vi "(Incomplete) Beta Function (obs).vi"(3 "a":dbl=nan format="%.2f", 4 "y":dbl format="%.2f", 5 "x":dbl format="%.2f") -> (2 "b(x, y, a)":dbl format="%.2f")   [LabVIEW 2020, in "NI_Gmath.lvlib"]
uses:
  NI_Gmath.lvlib
panel:
  # "This VI is obsolete !!!\nYou should replace this VI in your diagram with the \n(Incomplete) Beta Function VI.\n\nNOTE:   Please be aware that the new (Incomplete) Beta\n             Function VI is a polymorphic VI. If you leave the a\n             input of this obsolete VI unwired, please use the \n             Beta Function instance of the new (Incomplete)\n             Beta Function VI."
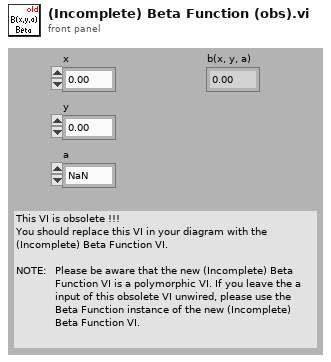
[diagram p1: front panel]
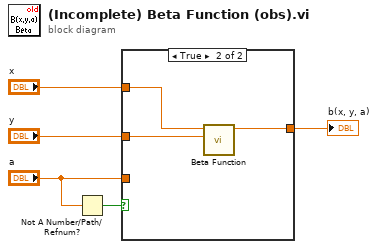
[diagram p0: block diagram]
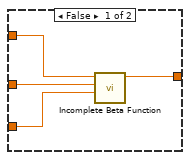
[diagram p2: hidden frame]
diagram:
  n1 = Not A Number/Path/Refnum?(number/path/refnum="a") -> (NaN/Path/Refnum?=w5:bool)
  n2 = case shown="True" w5 {
    tunnel: "x" -> [w9 w12]
    tunnel: "y" -> [w8 w11]
    tunnel: [w6 w10] -> w1
    tunnel: "a" -> [w7 _]
    frame False {
      n3 = call "Incomplete Beta Function.vi"("a"=w7, "y"=w8, "x"=w9) -> ("b(x, y, a)"=w6:dbl)  [unwired: 8 in]
    }
    frame True {
      n4 = call "Beta Function.vi"("y"=w11, "x"=w12) -> ("b(x, y)"=w10:dbl)  [unwired: 9 in]
    }
  }
  "b(x, y, a)" <- w1
